vi "wireframe.vi"() -> ()   [LabVIEW 2015, in "lv-blog-interface-prototype.lvlib"]
uses:
  lv-blog-interface-prototype.lvlib
panel:
  in  "tab_control":enum32{"Tool", "Build"}(tab)
  # "Project"
  # "Version"
  # "Git Commit Hash"
  # "Status"
  # "Tool (Navigation)"
  # "Build (Navigation)"
  # "Exit"
  # "Select Project"
  # "Configure"
  # "Depenencies"
  # "Open Dist Folder"
  # "Load Class"
  # "Exit"
  # "This space should be filled with something, possibly a general \"how to\" and some explanation in lieu of a help button? This may be an opportunity to add a logo if branding is desired"
  # "Configure Build"
  # "Possible Build Artifacts (tree)"
  # "P\nr\no\ng\nr\ne\ns\ns"
  # "Build"
  # "Post"
  # "Start"
  # "Cancel"
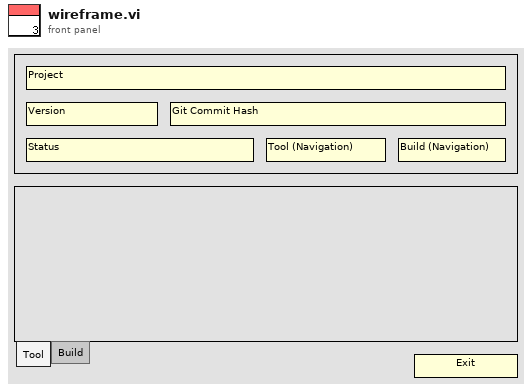
[diagram p1: front panel]
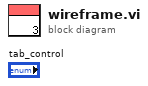
[diagram p0: block diagram]
diagram:
